vi "Calculate Gain.vi"(1 "Average Input Power (dBm)":dbl, 4 "Average Output Power (dBm)":dbl) -> (0 "Gain (dB)":dbl)   [LabVIEW 2016, in "RDLUtilities.lvlib"]
uses:
  RDLUtilities.lvlib
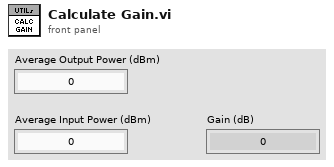
[diagram p1: front panel]
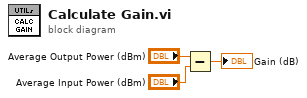
[diagram p0: block diagram]
diagram:
  n1 = Subtract(x="Average Output Power (dBm)", y="Average Input Power (dBm)") -> (x-y=→"Gain (dB)":dbl)
